vi "Gestion timing_Ligne 1.vi"(9 "L1 in":T1 {"t0" format="%<%.3X>T"}, 11 "Queue in":refnum<queue>) -> (1 "L1 out":T1 {"t0" format="%<%.3X>T"})   [LabVIEW 2014, in "PLS Digital Control.lvlib"]
uses:
  PLS Digital Control.lvlib
  support/Message Queue/Message Cluster.ctl
  support/Message Queue/Enqueue Message (Single).vi
  support/Message Queue/PLS Message Queue.lvlib
panel:
  out "Elapsed Time (s)":dbl
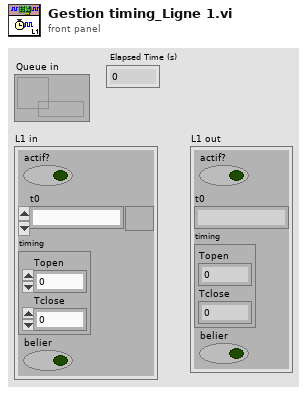
[diagram p1: front panel]
types:
  T1 = cluster{"actif?":bool, "t0":timestamp, "timing":cluster{"Topen":dbl, "Tclose":dbl}, "belier":bool}
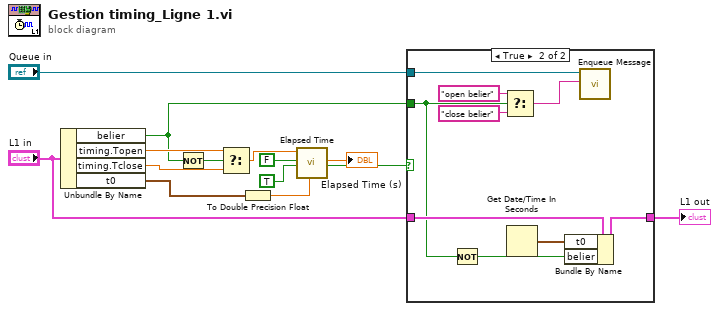
[diagram p0: block diagram]
diagram:
  n1 = Unbundle By Name("L1 in") -> ("belier"=w4:bool, "timing.Topen"=w7:dbl, "timing.Tclose"=w6:dbl, "t0"=w8:timestamp)
  n2 = Not(x=w4) -> (.not. x?=w5:bool)
  n3 = Select(t=w7, s=w5, f=w6) -> (s? t:f=w1:dbl)
  n4 = To Double Precision Float(number=w8) -> (double precision float=w11:dbl)
  n5 = call "Elapsed Time"("Time Target (s)"=w1, "Reset"=FALSE, "Auto Reset"=TRUE, "Set Start Time (s)"=w11) -> ("Elapsed Time (s)"=→"Elapsed Time (s)":dbl, "Time has Elapsed"=w10:bool)  [unwired: 8 in, 6 out]
  n6 = case shown="True" w10 {
    tunnel: "Queue in" -> [_ w24]
    tunnel: w4 -> [_ w17]
    tunnel: "L1 in" -> [w15 w20]
    tunnel: [w15 w19] -> w2
    frame False {
    }
    frame True {
      n7 = Not(x=w17) -> (.not. x?=w16:bool)
      n8 = Select(t="open belier" ("Message"), s=w17, f="close belier" ("Message")) -> (s? t:f=w22:string)
      n9 = Get Date/Time In Seconds() -> (seconds since 1Jan1904=w18:timestamp)
      n10 = Bundle By Name(cluster=w20, "t0"=w18, "belier"=w16) -> (w19:T1)
      n11 = call-poly "Enqueue Message.vi"("Message"=w22, "Message Queue"=w24) -> ()  [unwired: 8 in, 2 out]
    }
  }
  "L1 out" <- w2
